vi "Process Outgoing Messages.vi"(0 "internal data":T1={"J1939 XNET Settings"={"XNET Database"="", "XNET Cluster"="", "CAN port"="", "Baud rate [Bd]"=0, "J1939 Network Address"=0, "Name"=0, "Termination"=0}, "j1939 queues"={"Processed Outgoing"=refnum, "Process Outgoing"=refnum, "stop notifier"=refnum, "error queue"=refnum, "active dtc"=refnum, "processed inc"=refnum}, "fgv references"={"BAM Buffer"=refnum, "CM Buffer"=refnum, "CM Gen"=refnum, "BAM Gen"=refnum, "Address Claims"=refnum, "RQST"=refnum, "scaling lut"=refnum, "data lut"=refnum, "cyclic scheduler"=refnum}, "frame in"="", "frame out"="", "timing"={"tb to j1939 queue timeout"=100, "j1939 to tb queue timeout"=100, "dtc loop period (ms)"=100, "CAN in loop period (ms)"=100, "process incoming queue timeout (ms)"=100, "Outgoing Write Decimation"=0, "process outgoing loop rate (ms)"=0, "periodic outgoing queue timeout (ms)"=10, "CAN out queue timeout (ms)"=100}}, 11 "error in":errorcluster, 12 "timeout in ms (-1)":i32=10) -> (4 "internal data out":T1={"J1939 XNET Settings"={"XNET Database"="", "XNET Cluster"="", "CAN port"="", "Baud rate [Bd]"=0, "J1939 Network Address"=0, "Name"=0, "Termination"=0}, "j1939 queues"={"Processed Outgoing"=refnum, "Process Outgoing"=refnum, "stop notifier"=refnum, "error queue"=refnum, "active dtc"=refnum, "processed inc"=refnum}, "fgv references"={"BAM Buffer"=refnum, "CM Buffer"=refnum, "CM Gen"=refnum, "BAM Gen"=refnum, "Address Claims"=refnum, "RQST"=refnum, "scaling lut"=refnum, "data lut"=refnum, "cyclic scheduler"=refnum}, "frame in"="", "frame out"="", "timing"={"tb to j1939 queue timeout"=100, "j1939 to tb queue timeout"=100, "dtc loop period (ms)"=100, "CAN in loop period (ms)"=100, "process incoming queue timeout (ms)"=100, "Outgoing Write Decimation"=0, "process outgoing loop rate (ms)"=0, "periodic outgoing queue timeout (ms)"=10, "CAN out queue timeout (ms)"=100}}, 13 "Message Errors":errorcluster, 15 "error out":errorcluster)   [LabVIEW 2013, in "J1939.lvlib"]
uses:
  J1939.lvlib
  API Types/Internal Data.ctl
  API Types/XNET Settings.ctl
  API Types/Setup Information Cluster.ctl
  API Types/CAN Outgoing Message Cluster.ctl
  API Types/Convert DTCs Cluster.ctl
  <vilib>/xnet/xnet.llb/XNET Frame CAN.ctl
  <vilib>/xnet/xnet.llb/XNET Frame Type CAN.ctl
  TP/TP List References.ctl
  BAM/BAM Buffer Connections List_Ref.ctl
  Connection Mode/Connection Mode Generation Connection Ref.ctl
  BAM/BAM Generation Connections List_Ref.ctl
  LUTs/J1939 Address Table Reference.ctl
  RQST/RQST Lookup Table Reference.ctl
  LUTs/J1939 Conversion Lookup Table Reference.ctl
  LUTs/J1939 Data Lookup Table Reference.ctl
  LUTs/Cyclic Frame Scheduler Lut Reference.ctl
  Configuration/TypeDefs/timing configuration.ctl
  Check Output Message Frame Type.vi
  BAM/BAM Generation.vi
  BAM/BAM Generation Connections List_Actions.vi
  BAM/BAM Generation Create New TP Connection.vi
  Connection Mode/Connection Mode Generation.vi
  Connection Mode/Connection Mode Generation Connections List_Actions.vi
  Connection Mode/Connection Mode Generation Search for Connection (Local Message).vi
  Connection Mode/Connection Mode Generation Create New TP Connection.vi
  Convert Signals to Frame by ID.vi
  Frame Conversion/Common Conversions.vi
  Frame Conversion/Convert CAN Arb ID to J1939 ID.vi
  Common Messages/J1939 Common Messages.vi
  Common Messages/J1939 Message TP.CM BAM.vi
  Common Messages/J1939 Message TP.DT.vi
  Common Messages/J1939 Message TP.CM RTS.vi
  Conversion Lookup Table Get Conversion Parameter.vi
  LUTs/J1939 Data Lookup Table Get Signals (Range).vi
  Frame Conversion/Convert J1939 ID to CAN Arb ID.vi
  LUTs/Call Scheduler LUT.vi
  <vilib>/xnet/xnet.llb/XNET Convert.vi
  <vilib>/xnet/xnet.llb/XNET Convert (Signal to Frame Raw).vi
  BAM/BAM Generation Search for Connection (Local Message).vi
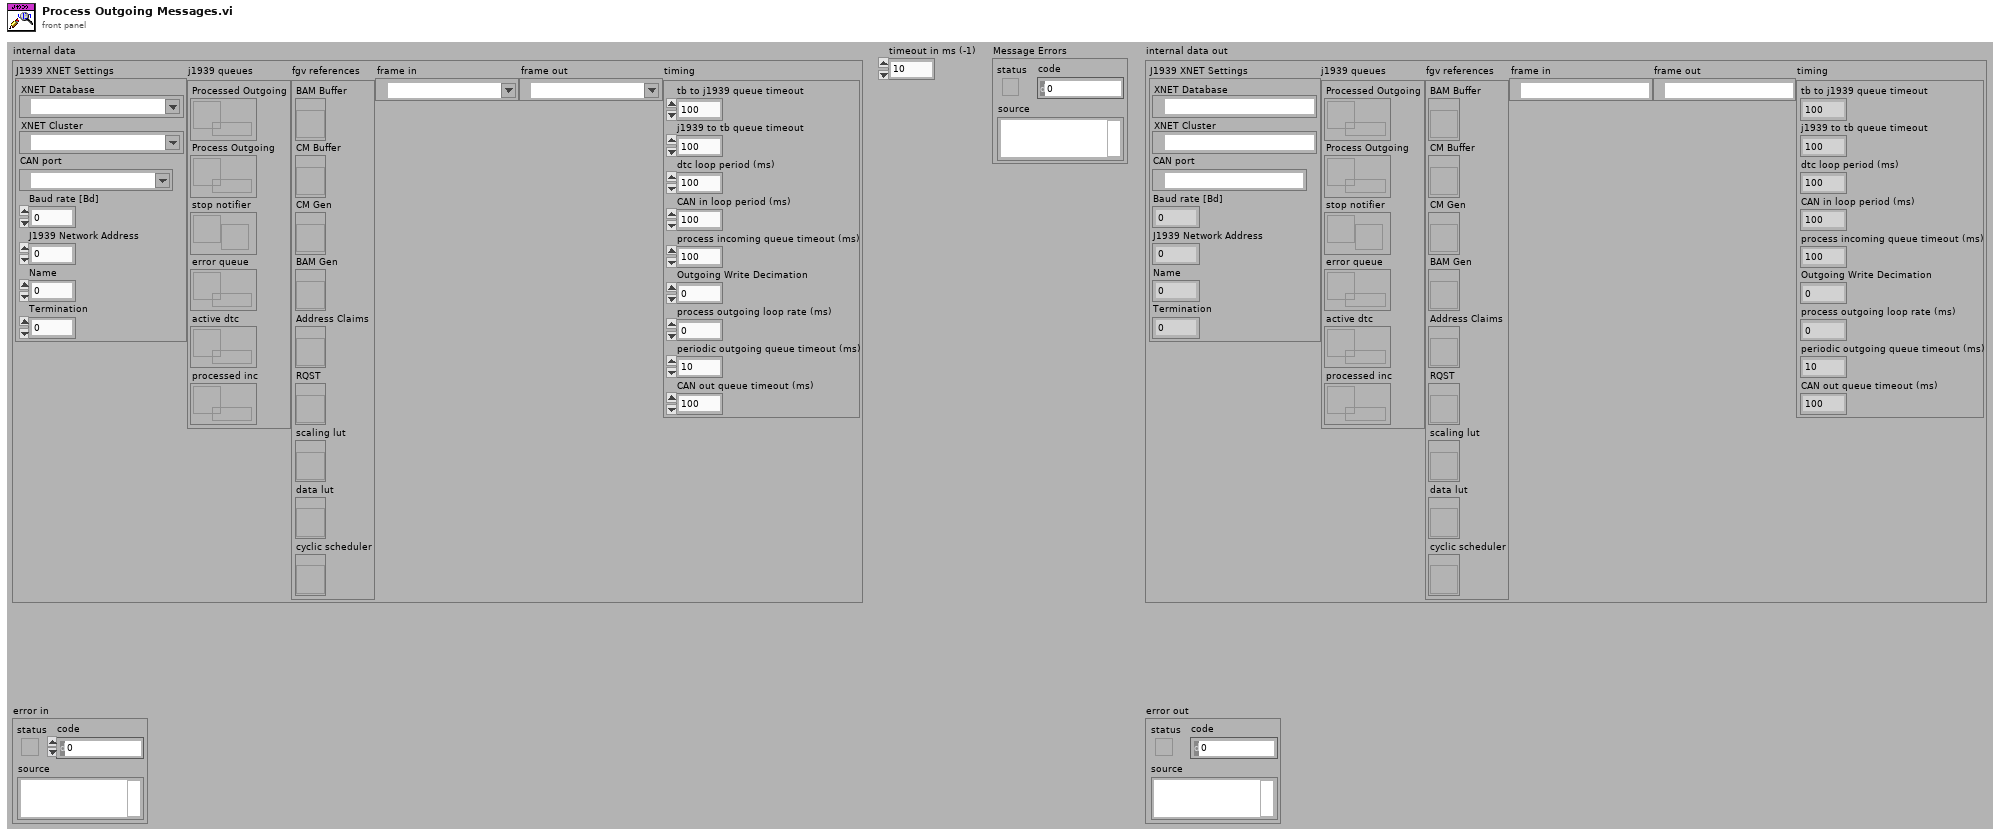
[diagram p1: front panel]
types:
  T1 = typedef "J1939.lvlib/Internal Data.ctl" = cluster{"J1939 XNET Settings":T2, "j1939 queues":T3, "fgv references":T4, "frame in":refnum<k21>, "frame out":refnum<k21>, "timing":T13}
  T2 = typedef "J1939.lvlib/XNET settings.ctl" = cluster{"XNET Database":refnum<k21>, "XNET Cluster":refnum<k21>, "CAN port":refnum<k21>, "Baud rate [Bd]":u32, "J1939 Network Address":u8, "Name":u64, "Termination":u32}
  T3 = typedef "J1939.lvlib/Setup Information Cluster.ctl" = cluster{"Processed Outgoing":refnum<queue>, "Process Outgoing":refnum<queue>, "stop notifier":refnum<notifier>, "error queue":refnum<queue>, "active dtc":refnum<queue>, "processed inc":refnum<queue>}
  T4 = typedef "J1939.lvlib/TP List References.ctl" = cluster{"BAM Buffer":T5, "CM Buffer":T5, "CM Gen":T6, "BAM Gen":T7, "Address Claims":T8, "RQST":T9, "scaling lut":T10, "data lut":T11, "cyclic scheduler":T12}
  T5 = typedef "J1939.lvlib/BAM Buffer Connections List_Ref.ctl" = refnum<vi>
  T6 = typedef "J1939.lvlib/Connection Mode Generation Connection Ref.ctl" = refnum<vi>
  T7 = typedef "J1939.lvlib/BAM Generation Connections List_Ref.ctl" = refnum<vi>
  T8 = typedef "J1939.lvlib/J1939 Address Table Reference.ctl" = refnum<vi>
  T9 = typedef "J1939.lvlib/RQST Lookup Table Reference.ctl" = refnum<vi>
  T10 = typedef "J1939.lvlib/J1939 Conversion Lookup Table Reference.ctl" = refnum<vi>
  T11 = typedef "J1939.lvlib/J1939 Data Lookup Table Reference.ctl" = refnum<vi>
  T12 = typedef "J1939.lvlib/cyclic frame scheduler lut reference.ctl" = refnum<vi>
  T13 = typedef "J1939.lvlib/timing configuration.ctl" = cluster{"tb to j1939 queue timeout":i32, "j1939 to tb queue timeout":i32, "dtc loop period (ms)":i32, "CAN in loop period (ms)":i32, "process incoming queue timeout (ms)":i32, "Outgoing Write Decimation":u32, "process outgoing loop rate (ms)":i32, "periodic outgoing queue timeout (ms)":i32, "CAN out queue timeout (ms)":i32}
  T14 = typedef "J1939.lvlib/CAN Outgoing Message Cluster.ctl" = cluster{"Identifier":u32, "Data":u8[]}
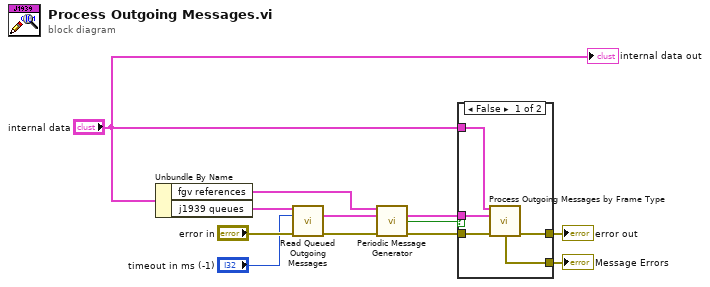
[diagram p0: block diagram]
diagram:
  n1 = Unbundle By Name("internal data") -> ("fgv references"=w2:T4, "j1939 queues"=w3:T3)
  n2 = call "Read Queued Outgoing Messages.vi"("j1939 queues"=w3, "timeout in ms (-1)"="timeout in ms (-1)", "error in"="error in") -> ("Output Array"=w8:T14[], "error out"=w10:errorcluster)  [unwired: 2 in, 9 out]
  n3 = call "Periodic Message Generator.vi"("fgv references"=w2, "Output Array"=w8, "error in"=w10) -> ("Output Array"=w7:T14[], "Empty?"=w6:bool, "error out"=w9:errorcluster)  [unwired: 4 in, 6 out]
  n4 = case shown="False" w6 {
    tunnel: [w17 w18] -> w11
    tunnel: w7 -> [w16 _]
    tunnel: w9 -> [w15 w18]
    tunnel: [w14 _] -> w5
    tunnel: "internal data" -> [w13 _]
    frame False {
      n5 = call "Process Outgoing Messages by Frame Type.vi"("internal data"=w13, "Output Array"=w16, "error in"=w15) -> ("Message Errors"=w14:errorcluster, "System Error"=w17:errorcluster)  [unwired: 1 in, 10 out]
    }
    frame True {
    }
  }
  "error out" <- w11
  "Message Errors" <- w5
  "internal data out" <- "internal data"
